vi "Set Workspace Color.vi"(8 "Error In":errorcluster, 11 "Color to set":u32(colorbox)) -> (0 "Error Out":errorcluster)   [LabVIEW 2013]
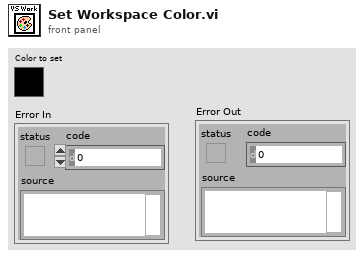
[diagram p1: front panel]
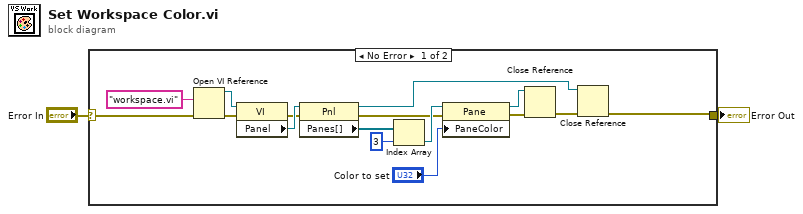
[diagram p0: block diagram]
diagram:
  n1 = case shown="No Error" "Error In" {
    selector: "Error In" -> [w11 w19]
    tunnel: [w3 w19] -> w1
    frame No Error {
      n2 = Open VI Reference(vi path="workspace.vi", error in (no error)=w11) -> (vi reference=w14:refnum<vi>, error out=w13:errorcluster)  [unwired: 4 in]
      n3 = property class="VI"(reference=w14, error in=w13) -> (error out=w10:errorcluster, "Panel"=w15:refnum<vi>)  [unwired: 1 out]
      n4 = property class="Pnl"(reference=w15, error in=w10) -> (reference out=w4:refnum<vi>, error out=w9:errorcluster, "Panes[]"=w16:refnum<vi>[])
      n5 = Index Array(array=w16, index=3) -> (element=w18:refnum<vi>)
      n6 = property class="Pane"(reference=w18, error in=w9, "PaneColor"="Color to set") -> (reference out=w6:refnum<vi>, error out=w7:errorcluster)
      n7 = Close Reference(reference=w6, error in (no error)=w7) -> (error out=w5:errorcluster)
      n8 = Close Reference(reference=w4, error in (no error)=w5) -> (error out=w3:errorcluster)
    }
    frame Error {
    }
  }
  "Error Out" <- w1
